vi "K2000_fetch_value.vi"(0 "ResourceNameIn":string="0:17", 7 "error in":errorcluster caption="entrée d'erreur" {"code" format="%.0x"}) -> (26 "token":dbl, 27 "error out":errorcluster caption="sortie d'erreur" {"code" format="%.0x"})   [LabVIEW 2013]
doc: "Launches the Instrument I/O Assistant, which you can use to communicate with message-based instruments and graphically parse the response. For example you can communicate with an instrument that uses a serial, Ethernet, or GPIB interface."
panel:
  out "String":string
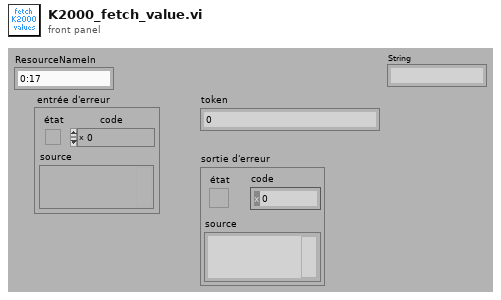
[diagram p1: front panel]
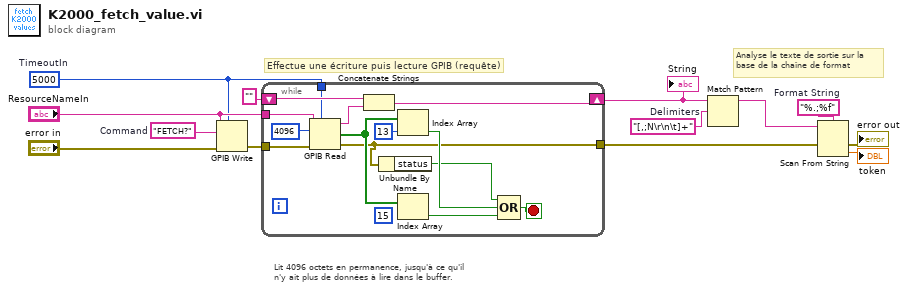
[diagram p0: block diagram]
diagram:
  w1 = "[,;N\r\n\t]+"  # Delimiters
  w4 = "%.;%f"  # Format String
  w10 = "FETCH?"  # Command
  w7 = 5000  # TimeoutIn
  # "Analyse le texte de sortie sur la base de la chaîne de format"
  # "Effectue une écriture puis lecture GPIB (requête)"
  # "Lit 4096 octets en permanence, jusqu'à ce qu'il\nn'y ait plus de données à lire dans le buffer."
  n1 = GPIB Write(0:"ResourceNameIn", 1:w10, 3:"error in", 4:w7) -> (6:w9:errorcluster)  [unwired: 1 in, 1 out]
  n2 = while {
    shift-right: [w26] -> w6
    shift-left: "" -> [w27]
    tunnel: w9 -> [w24]
    tunnel: [w15] -> w12
    tunnel: "ResourceNameIn" -> [w22]
    tunnel: w7 -> [w23]
    stop <- w17 stop-if-true
    (unwired) 15 ("index")
    n3 = GPIB Read(0:w22, 1:u32 4096 ("byte count (0)"), 3:w24, 4:w23) -> (5:w25:string, 6:w19:bool[], 7:w15:errorcluster)  [unwired: 1 out]
    n4 = Concatenate Strings(w27, w25) -> (w26:string)
    n5 = Unbundle By Name(w15) -> ("status"=w14:bool)
    n6 = Index Array(array=w19, index=13) -> (element=w18:bool)
    n7 = Index Array(array=w19) -> (element=w16:bool)  [unwired: 1 in]
    n8 = Compound Arithmetic op=OR(w14, w18, w16) -> (w17:bool)
  }
  "String" <- w6
  n9 = Match Pattern(string=w6, regular expression=w1) -> (before substring=w5:string)  [unwired: 4 out]
  n10 = Scan From String(format string=w4, input string=w5, error in=w12) -> (error out=→"error out":errorcluster, output 1=→"token":dbl)  [unwired: 1 in, 3 out]
